vi "MAIN VI - Separate text by style.vi"(11 "Text":string="Il était une fois un <b>jongleur qui ne <i>savait pas</i> jongler alors<u> il utilisa</b> un </u>arc.  Il demeurait quand même un <s>peu</s> suspicieux.  Il était une fois un <b>jongleur qui ne <i>savait pas</i> jongler alors<u> il utilisa</b> un </u>arc.  Il demeurait quand même un <s>peu</s> suspicieux.  Il était une fois un <b>jongleur qui ne <i>savait pas</i> jongler alors<u> il utilisa</b> un </u>arc.  Il demeurait quand même un <s>peu</s> suspicieux.") -> ()   [LabVIEW 2019, in "Exaprom PDF.lvlib"]
doc: "Version 1.0\nDeveloped by Jean-Marc Simard\nCopyright © 2010, Exaprom Inc.\nAll rights reserved.\nLicense: BSD"
uses:
  Exaprom PDF.lvlib
panel:
  out "msec3":u32
  out "msec2":u32
  out "msec1":u32=1
  out "msec tot":u32=1
  out "error out":errorcluster
  in  "error in (no error)":errorcluster
  out "Style and text [ ]":T1(array[cluster])
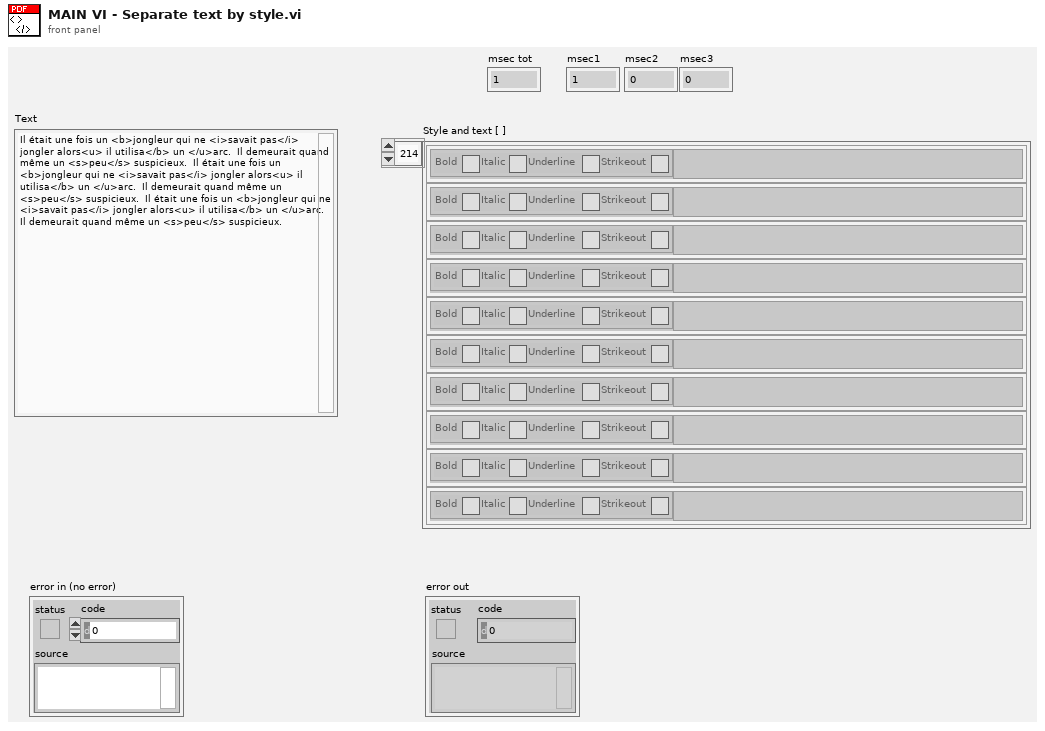
[diagram p1: front panel]
types:
  T1 = cluster{"Style":cluster{"Bold":bool, "Italic":bool, "Underline":bool, "Strikeout":bool}, "Text 2":string}[]
  T2 = typedef "Exaprom PDF.lvlib/HTML tags.ctl" = enum16{"N", "b", "u", "s", "i"}
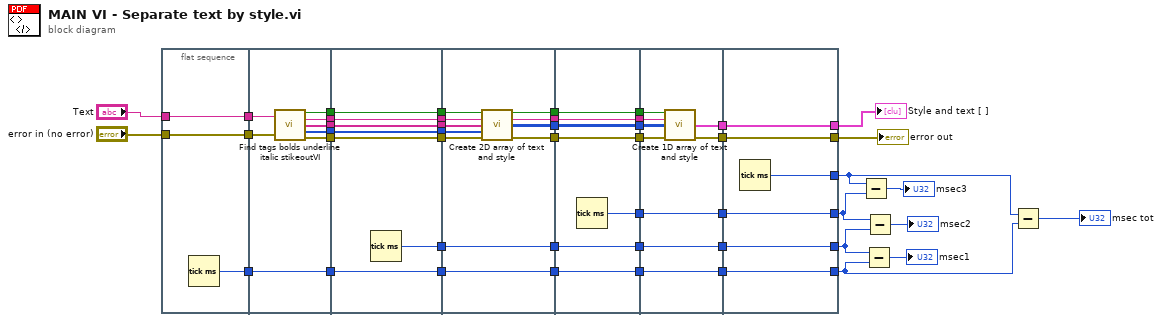
[diagram p0: block diagram]
diagram:
  n1 = flat-sequence {
    tunnel: "error in (no error)" -> [w48]
    tunnel: "Text" -> [w49]
    tunnel: [w49] -> w38
    tunnel: [w48] -> w37
    tunnel: [w47] -> w36
    tunnel: w38 -> [w56]
    tunnel: w37 -> [w55]
    tunnel: w36 -> [w57]
    tunnel: [w57] -> w32
    tunnel: [w54] -> w31
    tunnel: [w53] -> w28
    tunnel: [w52] -> w26
    tunnel: [w51] -> w25
    tunnel: [w50] -> w22
    tunnel: w32 -> [w64]
    tunnel: [w64] -> w35
    tunnel: w31 -> [w63]
    tunnel: [w63] -> w30
    tunnel: [w62] -> w29
    tunnel: w28 -> [w62]
    tunnel: [w61] -> w27
    tunnel: w26 -> [w61]
    tunnel: w25 -> [w60]
    tunnel: [w60] -> w24
    tunnel: [w59] -> w23
    tunnel: w22 -> [w59]
    tunnel: [w58] -> w10
    tunnel: w35 -> [w75]
    tunnel: [w75] -> w34
    tunnel: w30 -> [w74]
    tunnel: w29 -> [w73]
    tunnel: w27 -> [w72]
    tunnel: w24 -> [w71]
    tunnel: w23 -> [w70]
    tunnel: [w69] -> w20
    tunnel: [w68] -> w18
    tunnel: [w67] -> w16
    tunnel: [w66] -> w14
    tunnel: [w65] -> w11
    tunnel: w10 -> [w65]
    tunnel: w34 -> [w82]
    tunnel: [w82] -> w33
    tunnel: [w81] -> w21
    tunnel: w20 -> [w81]
    tunnel: [w80] -> w19
    tunnel: w18 -> [w80]
    tunnel: [w79] -> w17
    tunnel: w16 -> [w79]
    tunnel: [w78] -> w15
    tunnel: w14 -> [w78]
    tunnel: [w77] -> w12
    tunnel: w11 -> [w77]
    tunnel: [w76] -> w8
    tunnel: [w91] -> w42
    tunnel: [w90] -> w41
    tunnel: w33 -> [w89]
    tunnel: [w89] -> w40
    tunnel: w21 -> [w88]
    tunnel: w19 -> [w87]
    tunnel: w17 -> [w86]
    tunnel: w15 -> [w85]
    tunnel: [w84] -> w13
    tunnel: w12 -> [w84]
    tunnel: [w83] -> w9
    tunnel: w8 -> [w83]
    tunnel: [w96] -> w43
    tunnel: [w97] -> w45
    tunnel: w42 -> [w97]
    tunnel: w41 -> [w96]
    tunnel: w40 -> [w95]
    tunnel: [w95] -> w1
    tunnel: [w94] -> w2
    tunnel: [w93] -> w7
    tunnel: w13 -> [w93]
    tunnel: [w92] -> w6
    tunnel: w9 -> [w92]
    frame #0 {
      n2 = Tick Count (ms)() -> (millisecond timer value=w47:u32)
    }
    frame #1 {
      n3 = call "Find tags bolds underline italic stikeoutVI.vi"("Text"=w56, "error in (no error)"=w55) -> ("Find tag ?"=w54:bool, "Text out"=w53:string, "Tags list [ ]"=w52:string[], "Tags position [ ]"=w51:i32[], "error out"=w50:errorcluster)  [unwired: 9 out]
    }
    frame #2 {
      n4 = Tick Count (ms)() -> (millisecond timer value=w58:u32)
    }
    frame #3 {
      n5 = call "Create 2D array of text and style.vi"("Find tag ?"=w74, "Text"=w73, "Tags list [ ]"=w72, "Tags position [ ]"=w71, "error in (no error)"=w70) -> ("Find tag ? duplicate"=w69:bool, "Text duplicate"=w68:string, "Style [ ]"=w67:T2[][], "error out"=w66:errorcluster)  [unwired: 7 out]
    }
    frame #4 {
      n6 = Tick Count (ms)() -> (millisecond timer value=w76:u32)
    }
    frame #5 {
      n7 = call "Create 1D array of text and style.vi"("Find tag ?"=w88, "Text duplicate"=w87, "Style [ ]"=w86, "error in (no error)"=w85) -> ("Style and text [ ]"=w91:T1, "error out"=w90:errorcluster)  [unwired: 10 out]
    }
    frame #6 {
      n8 = Tick Count (ms)() -> (millisecond timer value=w94:u32)
    }
  }
  n9 = Subtract(x=w2, y=w6) -> (x-y=→"msec3":u32)
  n10 = Subtract(x=w7, y=w1) -> (x-y=→"msec1":u32)
  n11 = Subtract(x=w6, y=w7) -> (x-y=→"msec2":u32)
  n12 = Subtract(x=w2, y=w1) -> (x-y=→"msec tot":u32)
  "Style and text [ ]" <- w45
  "error out" <- w43
